vi "Fill From Zero Slider.vi"(1 "Numeric":dbl format="%#_6p") -> (0 "Slide 1":cluster{dbl, dbl}(slide)={0.0, -0.3030303030303032} scale=-10.0..10.0 scale format="%#_6p")   [LabVIEW 2016, in "SR7270 UI.lvclass"]
uses:
  SR7270 UI.lvclass
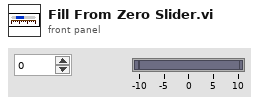
[diagram p1: front panel]
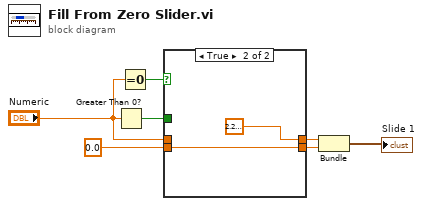
[diagram p0: block diagram]
diagram:
  n1 = Greater Than 0?(x="Numeric") -> (x > 0?=w6:bool)
  n2 = Equal To 0?(x="Numeric") -> (x = 0?=w2:bool)
  n3 = case shown="True" w2 {
    tunnel: w6 -> [w12 _]
    tunnel: [w11 2.220446049250313e-16] -> w5
    tunnel: "Numeric" -> [w10 _]
    tunnel: 0.0 ("Numeric") -> [w9 w18]
    tunnel: [w8 w18] -> w3
    frame False {
      n4 = case shown="False" w12 {
        tunnel: [w14 w16] -> w11
        tunnel: w10 -> [w13 w16]
        tunnel: w9 -> [w14 w15]
        tunnel: [w13 w15] -> w8
        frame False {
        }
        frame True {
        }
      }
    }
    frame True {
    }
  }
  n5 = Bundle("Numeric"=w5, "Numeric"=w3) -> (→"Slide 1":cluster{"Numeric":dbl, "Numeric":dbl})  [unwired: 1 in]
